vi "RT Loop watchdog.vi"(8 "error in":errorcluster, 11 "Watchdog pet rate (ms)":u32=1000) -> ()   [LabVIEW 2018]
uses:
  <vilib>/Platform/TimedLoop/XDataNode/timing_clust.ctl
  <vilib>/Platform/TimedLoop/XDataNode/nitl_modes.ctl
  <vilib>/Platform/TimedLoop/XDataNode/wakeup.ctl
  <vilib>/FPGAPlugInAG/cRIO-9074/niLvFpga_Open_cRIO-9074.vi
  <vilib>/rvi/interface/common/dynamic/niFpgaDynamicAddResources.vi
  <vilib>/Utility/error.llb/Error Cluster From Error Code.vi
  <vilib>/rvi/errors/niLvFpgaAdjustHostInterfaceError.vi
  <vilib>/rvi/interface/nirviOpenFPGA/nirviOpenFPGA.xnode
  FPGA Bitfiles/remotecontroller_FPGATarget_FPGAMain_RhGo+c1SRDI.lvbitx
  FPGA Main.vi
  <vilib>/rvi/interface/nirviReadWriteControl/nirviReadWriteControl.xnode
  <vilib>/Platform/TimedLoop/XDataNode/XDataNode.xnode
  NiFpgaLv.dll
  <vilib>/rvi/interface/Simulation/niFpgaSimulationCallBeginRW.vi
  <vilib>/Platform/TimedLoop/XDataNode/XDNodeRunTimeDep.lvlib
panel:
  out "number of pets":i32
  out "duration of iteration":i64
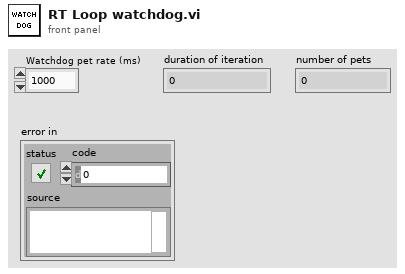
[diagram p1: front panel]
types:
  T1 = typedef "XDNodeRunTimeDep.lvlib/timing_clust.ctl" = cluster{"Expected End [f-1]":u64, "Actual End [f-1]":u64, "Finished Late? [f-1]":bool, "Expected End [i-1]":u64, "Actual End [i-1]":u64, "Finished Late? [i-1]":bool, "Expected Start [i]":u64, "Actual Start [i]":u64, "Expected Start [f]":u64, "Actual Start [f]":u64, "Source Name":string, "Structure Name":string, "Period":i64, "Deadline":i64, "Offset":i64, "Start":i64, "Priority":i32, "Timeout":i32, "Mode":T2, "Wakeup Reason":T3, "Error":errorcluster, "Source Type":string, "Secondary Source Type":string, "Global End Time":u64, "Global Start Time":u64, "Frame Duration":u64, "Iteration Duration":u64, "Assigned CPU":i32, "I/O Scan Engine Mode":u32}
  T2 = typedef "XDNodeRunTimeDep.lvlib/nitl_modes.ctl" = enum32{"No Change", "Process missed periods, maintain original phase", "Discard missed periods, maintain original phase", "Process missed periods, ignore original phase", "Discard missed periods, ignore original phase"}
  T3 = typedef "XDNodeRunTimeDep.lvlib/wakeup.ctl" = enum32{"Normal", "Aborted", "Asynchronous wakeup", "Timing source error", "Timed loop error", "Timeout"}
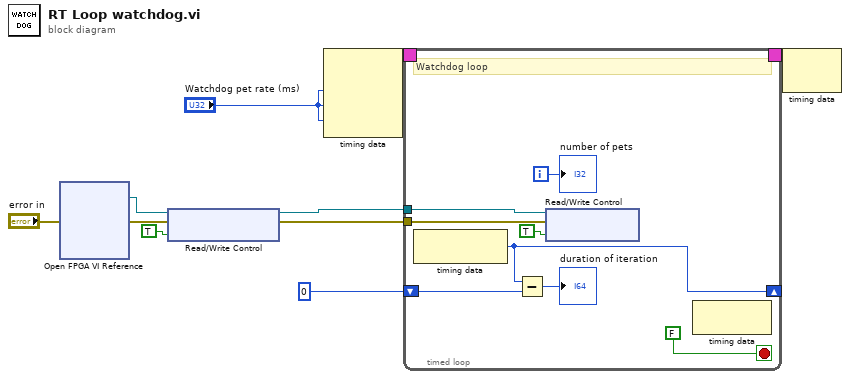
[diagram p0: block diagram]
diagram:
  n1 = xnode "Open FPGA VI Reference"("error in"="error in") -> ("FPGA VI Reference Out"=w10:refnum<k20>, "error out"=w9:errorcluster)  [unwired: 1 in]
  n2 = xnode "Read/Write Control"("FPGA VI Reference In"=w10, "error in"=w9, "Enable Watchdog"=TRUE) -> ("FPGA VI Reference Out"=w7:refnum<k20>, "error out"=w6:errorcluster)
  n3 = node-c288("Watchdog pet rate (ms)", "Watchdog pet rate (ms)", "Watchdog pet rate (ms)") -> (w4:T1)  [unwired: 1 in]
  n4 = timed-loop {
    tunnel: w7 -> [w18]
    tunnel: w6 -> [w17]
    timing: w4 -> [_]
    timing-out: [_] -> w3
    shift-right: [w12] -> _
    shift-left: i64 0 -> [w14]
    i -> [w16]
    stop <- FALSE stop-if-true
    # "Watchdog loop"
    n5 = node-c288() -> (w12:i64)  [unwired: 1 in]
    n6 = Subtract(x=w12, y=w14) -> (x-y=→"duration of iteration":i64)
    n7 = xnode "Read/Write Control"("FPGA VI Reference In"=w18, "error in"=w17, "Pet Watchdog"=TRUE) -> ()  [unwired: 2 out]
    n8 = node-c288() -> ()  [unwired: 1 in, 1 out]
    "number of pets" <- w16
  }
  n9 = node-c288(w3) -> ()  [unwired: 1 out]
